vi "Add Result.vi"(8 "Header":string="dCt", 9 "dCt":dbl[][](array[numeric]), 10 "RowHdrs Input":string[](array[string]), 11 "Input":string[][][](array[string])) -> (2 "RowHdrs Output":string[](array[string]), 3 "Output":string[][][](array[string]))   [LabVIEW 2017]
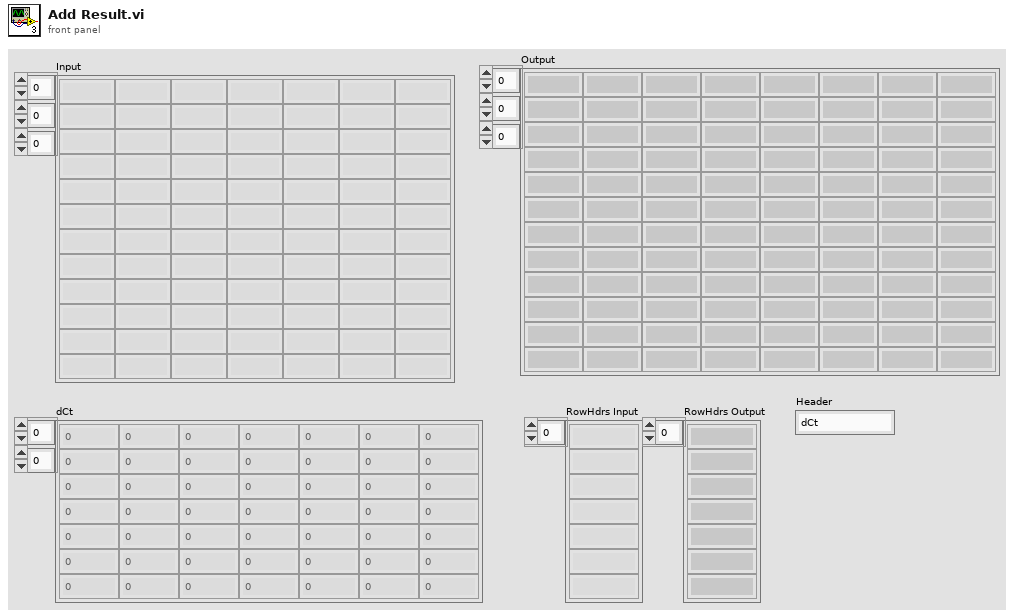
[diagram p1: front panel]
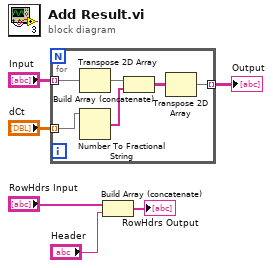
[diagram p0: block diagram]
diagram:
  n1 = for {
    tunnel: "Input" -> [w12] mode=indexing
    tunnel: "dCt" -> [w11] mode=indexing
    tunnel: [w7] -> w4 mode=indexing
    n2 = Transpose 2D Array(2D array=w12) -> (transposed array=w10:string[][])
    n3 = Number To Fractional String(number=w11) -> (F-format string=w9:string[])  [unwired: 3 in]
    n4 = Build Array (concatenate)(w10, w9) -> (w8:string[][])
    n5 = Transpose 2D Array(2D array=w8) -> (transposed array=w7:string[][])
  }
  "Output" <- w4
  n6 = Build Array (concatenate)("RowHdrs Input", "Header") -> (→"RowHdrs Output":string[])
